vi "Command Started.vi"(8 "error in (no error)":errorcluster, 10 "Command Name (Instance)":string, 11 "Command Processor Actor in":refnum<class "Command Processor Actor.lvclass">) -> (0 "error out":errorcluster, 3 "Command Processor Actor out":refnum<class "Command Processor Actor.lvclass">)   [LabVIEW 2014, in "Robot Actor Framework.lvlib" / "Command Processor Actor.lvlib" / "Command Processor Actor.lvclass"]
uses:
  Command Processor Actor.lvclass
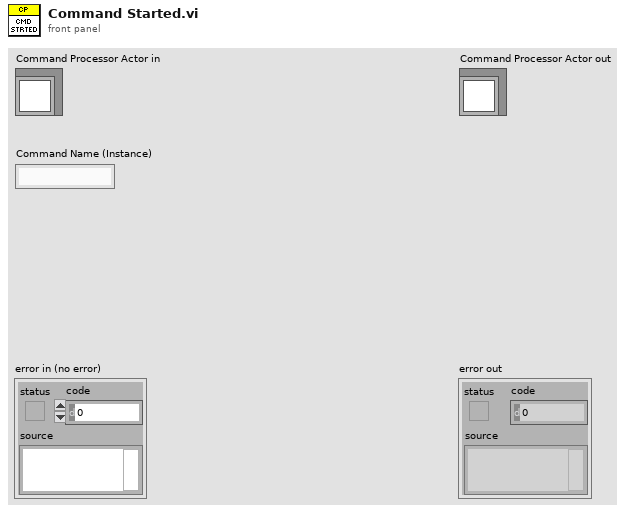
[diagram p1: front panel]
types:
  T1 = enum16{"Critical", "Error", "Warning", "Informational", "Debug"}
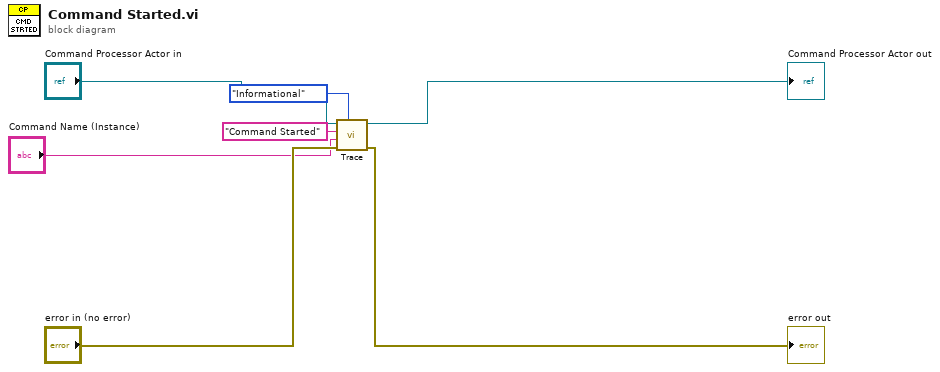
[diagram p0: block diagram]
diagram:
  n1 = call-dynamic "Trace.vi"("Trace Level"=T1."Informational", "error in (no error)"="error in (no error)", "Command Processor Message"="Command Name (Instance)", "Command Processor Action"="Command Started", "Command Processor Actor in"="Command Processor Actor in") -> ("error out"=→"error out":errorcluster, "Command Processor Actor out"=→"Command Processor Actor out":refnum<class "Command Processor Actor.lvclass">)  [unwired: 5 in]
